vi "Binary_Array_to_Decimal.vi"(11 "Array":i32[](array[numeric])) -> ()   [LabVIEW 2016]
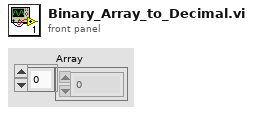
[diagram p1: front panel]
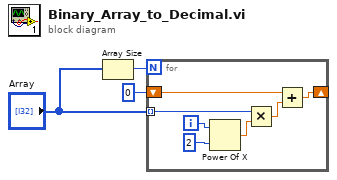
[diagram p0: block diagram]
diagram:
  n1 = Array Size(array="Array") -> (size(s)=w3:i32)
  n2 = for {
    N: w3 -> [_]
    tunnel: "Array" -> [w7] mode=indexing
    shift-right: [w4] -> _
    shift-left: 0 -> [w5]
    i -> [w9]
    n3 = Power Of X(1:2, 2:w9) -> (0:w8:dbl)
    n4 = Multiply(x=w7, y=w8) -> (x*y=w6:dbl)
    n5 = Add(x=w5, y=w6) -> (x+y=w4:dbl)
  }
